vi "General configuration ILD1420.vi"(0 "Target mode":string(combo)="STANDARD", 1 "Averaging mode":string(combo)="MEDIAN", 2 "Averaging depth":u16=9, 3 "Trigger mode":string(combo)="NONE", 4 "Hold last value on error":string(combo)="NONE", 5 "N samples to hold":u16=1, 6 "Signal peak mode":string(combo)="DISTA", 7 "Activate error output":string(combo)="DIST", 8 "Data rate (kHz)":string(combo)="0.25", 9 "Error output mode":string(combo)="NPN", 10 "COM port":refnum<visa-resource-name>) -> (19 "Error out":errorcluster)   [LabVIEW 2015]
panel:
  # "PN 12/08/2016"
  # "-- MOVING: Moving averaging value (averaging depth 2, 4, 8, 16, 32, 64 and 128 possible)\n-- RECURSIVE: Recursive averaging value (averaging depth 1 up to 32768 possible)\n-- MEDIAN: Median (averaging depth 3, 5, 7 and 9 possible)"
  # "-- DISTA: output of peak with highest amplitude\n-- DIST1: output of first peak\n-- DISTL: output of last peak"
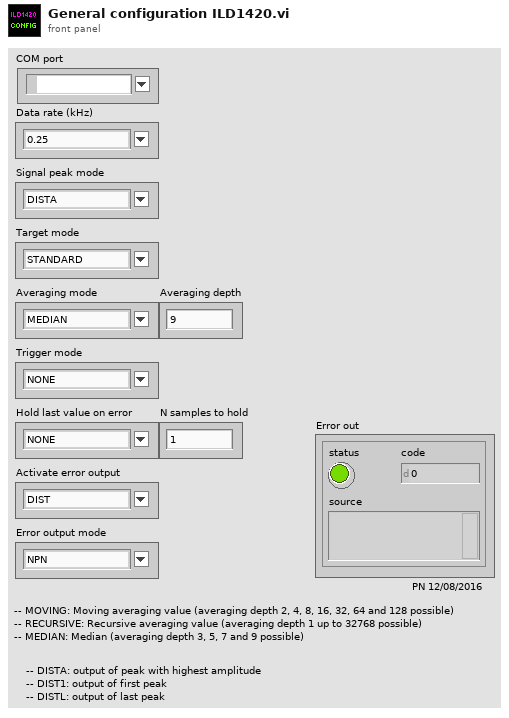
[diagram p1: front panel]
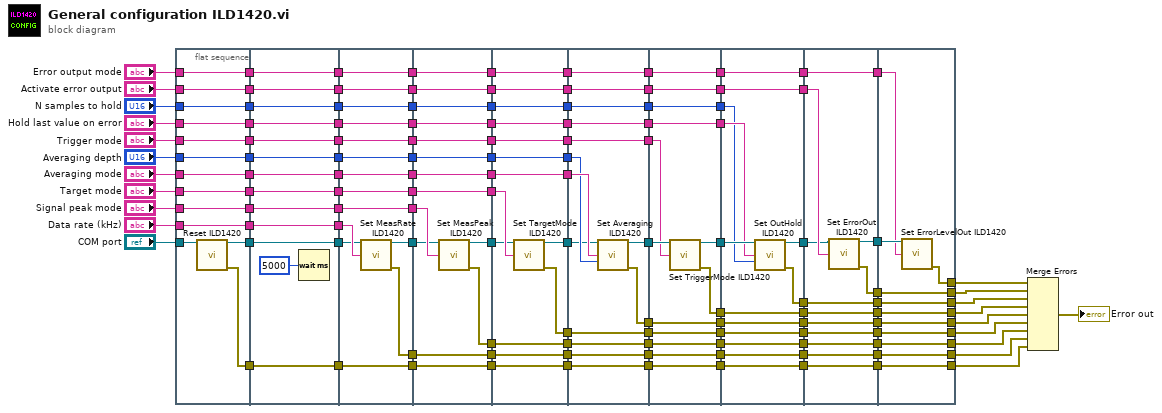
[diagram p0: block diagram]
diagram:
  n1 = flat-sequence {
    tunnel: "COM port" -> [w135]
    tunnel: [w135] -> w90
    tunnel: [w134] -> w88
    tunnel: "Data rate (kHz)" -> [w134]
    tunnel: [w133] -> w86
    tunnel: [w132] -> w84
    tunnel: "Signal peak mode" -> [w132]
    tunnel: "Target mode" -> [w131]
    tunnel: [w131] -> w82
    tunnel: "Averaging mode" -> [w130]
    tunnel: [w130] -> w80
    tunnel: "Averaging depth" -> [w129]
    tunnel: [w129] -> w78
    tunnel: "Trigger mode" -> [w128]
    tunnel: [w128] -> w44
    tunnel: "Hold last value on error" -> [w127]
    tunnel: [w127] -> w33
    tunnel: "N samples to hold" -> [w126]
    tunnel: [w126] -> w25
    tunnel: "Activate error output" -> [w125]
    tunnel: [w125] -> w15
    tunnel: "Error output mode" -> [w124]
    tunnel: [w124] -> w4
    tunnel: w90 -> [w148]
    tunnel: [w148] -> w89
    tunnel: w88 -> [w147]
    tunnel: [w147] -> w87
    tunnel: w86 -> [w146]
    tunnel: [w146] -> w85
    tunnel: w84 -> [w145]
    tunnel: [w145] -> w83
    tunnel: w82 -> [w144]
    tunnel: [w144] -> w81
    tunnel: w80 -> [w143]
    tunnel: [w143] -> w79
    tunnel: w78 -> [w142]
    tunnel: [w142] -> w77
    tunnel: [w140] -> w45
    tunnel: w44 -> [w140]
    tunnel: [w139] -> w34
    tunnel: w33 -> [w139]
    tunnel: [w138] -> w26
    tunnel: w25 -> [w138]
    tunnel: [w137] -> w16
    tunnel: w15 -> [w137]
    tunnel: [w136] -> w5
    tunnel: w4 -> [w136]
    tunnel: w89 -> [w158]
    tunnel: w87 -> [w161]
    tunnel: w85 -> [w159]
    tunnel: [w160] -> w121
    tunnel: [w159] -> w120
    tunnel: [w158] -> w119
    tunnel: w83 -> [w157]
    tunnel: [w157] -> w117
    tunnel: [w156] -> w110
    tunnel: w81 -> [w156]
    tunnel: [w155] -> w101
    tunnel: w79 -> [w155]
    tunnel: [w154] -> w97
    tunnel: w77 -> [w154]
    tunnel: [w153] -> w46
    tunnel: w45 -> [w153]
    tunnel: [w152] -> w35
    tunnel: w34 -> [w152]
    tunnel: [w151] -> w27
    tunnel: w26 -> [w151]
    tunnel: [w150] -> w17
    tunnel: w16 -> [w150]
    tunnel: [w149] -> w6
    tunnel: w5 -> [w149]
    tunnel: w121 -> [w174]
    tunnel: w120 -> [w172]
    tunnel: w119 -> [w170]
    tunnel: w117 -> [w171]
    tunnel: [w174] -> w116
    tunnel: [w173] -> w115
    tunnel: [w172] -> w114
    tunnel: [w170] -> w113
    tunnel: [w169] -> w111
    tunnel: w110 -> [w169]
    tunnel: [w168] -> w102
    tunnel: w101 -> [w168]
    tunnel: [w167] -> w98
    tunnel: w97 -> [w167]
    tunnel: [w166] -> w47
    tunnel: w46 -> [w166]
    tunnel: [w165] -> w36
    tunnel: w35 -> [w165]
    tunnel: [w164] -> w28
    tunnel: w27 -> [w164]
    tunnel: [w163] -> w18
    tunnel: w17 -> [w163]
    tunnel: [w162] -> w7
    tunnel: w6 -> [w162]
    tunnel: w116 -> [w187]
    tunnel: w115 -> [w186]
    tunnel: w114 -> [w185]
    tunnel: w113 -> [w182]
    tunnel: w111 -> [w183]
    tunnel: [w187] -> w109
    tunnel: [w186] -> w108
    tunnel: [w185] -> w107
    tunnel: [w184] -> w106
    tunnel: [w182] -> w105
    tunnel: [w181] -> w103
    tunnel: w102 -> [w181]
    tunnel: [w180] -> w99
    tunnel: w98 -> [w180]
    tunnel: [w179] -> w48
    tunnel: w47 -> [w179]
    tunnel: [w178] -> w37
    tunnel: w36 -> [w178]
    tunnel: [w177] -> w29
    tunnel: w28 -> [w177]
    tunnel: [w176] -> w19
    tunnel: w18 -> [w176]
    tunnel: [w175] -> w8
    tunnel: w7 -> [w175]
    tunnel: w109 -> [w200]
    tunnel: w108 -> [w199]
    tunnel: w107 -> [w198]
    tunnel: w106 -> [w197]
    tunnel: w105 -> [w193]
    tunnel: w103 -> [w195]
    tunnel: w99 -> [w194]
    tunnel: [w200] -> w76
    tunnel: [w199] -> w75
    tunnel: [w198] -> w74
    tunnel: [w197] -> w73
    tunnel: [w196] -> w72
    tunnel: [w193] -> w56
    tunnel: [w192] -> w49
    tunnel: w48 -> [w192]
    tunnel: [w191] -> w38
    tunnel: w37 -> [w191]
    tunnel: [w190] -> w30
    tunnel: w29 -> [w190]
    tunnel: [w189] -> w20
    tunnel: w19 -> [w189]
    tunnel: [w188] -> w9
    tunnel: w8 -> [w188]
    tunnel: w76 -> [w212]
    tunnel: w75 -> [w211]
    tunnel: w74 -> [w210]
    tunnel: w73 -> [w209]
    tunnel: w72 -> [w208]
    tunnel: [w212] -> w71
    tunnel: [w211] -> w70
    tunnel: [w210] -> w69
    tunnel: [w209] -> w68
    tunnel: [w208] -> w67
    tunnel: w56 -> [w207]
    tunnel: [w207] -> w55
    tunnel: [w206] -> w52
    tunnel: w49 -> [w205]
    tunnel: [w204] -> w39
    tunnel: w38 -> [w204]
    tunnel: [w203] -> w31
    tunnel: w30 -> [w203]
    tunnel: [w202] -> w21
    tunnel: w20 -> [w202]
    tunnel: [w201] -> w10
    tunnel: w9 -> [w201]
    tunnel: w71 -> [w224]
    tunnel: w70 -> [w223]
    tunnel: w69 -> [w222]
    tunnel: w68 -> [w221]
    tunnel: w67 -> [w220]
    tunnel: [w224] -> w66
    tunnel: [w223] -> w65
    tunnel: [w222] -> w64
    tunnel: [w221] -> w63
    tunnel: [w220] -> w62
    tunnel: w55 -> [w218]
    tunnel: [w219] -> w53
    tunnel: w52 -> [w219]
    tunnel: [w218] -> w43
    tunnel: [w217] -> w41
    tunnel: w39 -> [w216]
    tunnel: w31 -> [w215]
    tunnel: [w214] -> w22
    tunnel: w21 -> [w214]
    tunnel: [w213] -> w11
    tunnel: w10 -> [w213]
    tunnel: w66 -> [w235]
    tunnel: w65 -> [w234]
    tunnel: w64 -> [w233]
    tunnel: w63 -> [w232]
    tunnel: w62 -> [w231]
    tunnel: [w235] -> w61
    tunnel: [w234] -> w60
    tunnel: [w233] -> w59
    tunnel: [w232] -> w58
    tunnel: [w231] -> w57
    tunnel: [w230] -> w54
    tunnel: w53 -> [w230]
    tunnel: w43 -> [w226]
    tunnel: [w229] -> w42
    tunnel: w41 -> [w229]
    tunnel: [w228] -> w24
    tunnel: w22 -> [w227]
    tunnel: [w226] -> w14
    tunnel: [w225] -> w12
    tunnel: w11 -> [w225]
    tunnel: [w242] -> w96
    tunnel: [w243] -> w95
    tunnel: [w244] -> w92
    tunnel: [w245] -> w94
    tunnel: [w246] -> w93
    tunnel: w61 -> [w246]
    tunnel: w60 -> [w245]
    tunnel: w59 -> [w244]
    tunnel: w58 -> [w243]
    tunnel: w57 -> [w242]
    tunnel: [w241] -> w51
    tunnel: w54 -> [w241]
    tunnel: w42 -> [w240]
    tunnel: [w240] -> w3
    tunnel: [w239] -> w2
    tunnel: w24 -> [w239]
    tunnel: w14 -> [w238]
    tunnel: [w237] -> w1
    tunnel: w12 -> [w236]
    frame #0 {
      n2 = call "Reset ILD1420.vi"("COM port"=w135) -> ("Error out"=w133:errorcluster)  [unwired: 14 in]
    }
    frame #1 {
      n3 = Wait (ms)(milliseconds to wait=u32 5000) -> ()  [unwired: 1 out]
    }
    frame #2 {
      n4 = call "Set MeasRate ILD1420.vi"("COM port"=w158, "Data rate (kHz)"=w161) -> ("Error out"=w160:errorcluster)  [unwired: 13 in]
    }
    frame #3 {
      n5 = call "Set MeasPeak ILD1420.vi"("COM port"=w170, "Signal peak mode"=w171) -> ("Error out"=w173:errorcluster)  [unwired: 13 in]
    }
    frame #4 {
      n6 = call "Set TargetMode ILD1420.vi"("COM port"=w182, "Target mode"=w183) -> ("Error out"=w184:errorcluster)  [unwired: 13 in]
    }
    frame #5 {
      n7 = call "Set Averaging ILD1420.vi"("COM port"=w193, "Averaging mode"=w195, "Averaging depth"=w194) -> ("Error out"=w196:errorcluster)  [unwired: 12 in]
    }
    frame #6 {
      n8 = call "Set TriggerMode ILD1420.vi"("COM port"=w207, "Trigger mode"=w205) -> ("Error out"=w206:errorcluster)  [unwired: 13 in]
    }
    frame #7 {
      n9 = call "Set OutHold ILD1420.vi"("COM port"=w218, "Hold last value on error"=w216, "N samples to hold"=w215) -> ("Error out"=w217:errorcluster)  [unwired: 12 in]
    }
    frame #8 {
      n10 = call "Set ErrorOut ILD1420.vi"("COM port"=w226, "Activate error output"=w227) -> ("Error out"=w228:errorcluster)  [unwired: 13 in]
    }
    frame #9 {
      n11 = call "Set ErrorLevelOut ILD1420.vi"("COM port"=w238, "Error output mode"=w236) -> ("Error out"=w237:errorcluster)  [unwired: 13 in]
    }
  }
  n12 = Merge Errors(w1, w2, w3, w51, w96, w95, w94, w93, w92) -> (→"Error out":errorcluster)
